vi "Unescape String.vi"(11 "value":string) -> (3 "unescaped string":string)   [LabVIEW 2017, in "LVJSON.lvlib" / "JSON String.lvclass"]
uses:
  JSON String.lvclass
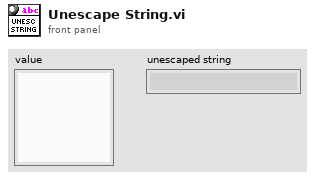
[diagram p1: front panel]
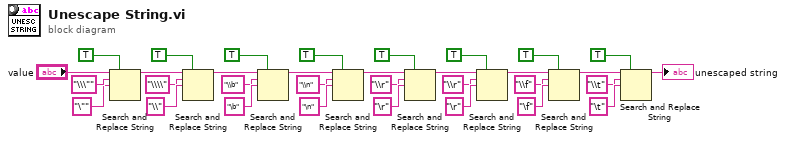
[diagram p0: block diagram]
diagram:
  n1 = Search and Replace String(replace all?=TRUE ("replace all? (F)"), input string="value", search string="\\\"" ("replace string (\"\")"), replace string="\"" ("search string")) -> (result string=w23:string)  [unwired: 4 in, 3 out]
  n2 = Search and Replace String(replace all?=TRUE ("replace all? (F)"), input string=w23, search string="\\\\" ("replace string (\"\")"), replace string="\\" ("search string")) -> (result string=w22:string)  [unwired: 4 in, 3 out]
  n3 = Search and Replace String(replace all?=TRUE ("replace all? (F)"), input string=w22, search string="\\b" ("replace string (\"\")"), replace string="\b" ("search string")) -> (result string=w29:string)  [unwired: 4 in, 3 out]
  n4 = Search and Replace String(replace all?=TRUE ("replace all? (F)"), input string=w29, search string="\\n" ("replace string (\"\")"), replace string="\n" ("search string")) -> (result string=w27:string)  [unwired: 4 in, 3 out]
  n5 = Search and Replace String(replace all?=TRUE ("replace all? (F)"), input string=w27, search string="\\r" ("replace string (\"\")"), replace string="\r" ("search string")) -> (result string=w25:string)  [unwired: 4 in, 3 out]
  n6 = Search and Replace String(replace all?=TRUE ("replace all? (F)"), input string=w25, search string="\\r" ("replace string (\"\")"), replace string="\r" ("search string")) -> (result string=w20:string)  [unwired: 4 in, 3 out]
  n7 = Search and Replace String(replace all?=TRUE ("replace all? (F)"), input string=w20, search string="\\f" ("replace string (\"\")"), replace string="\f" ("search string")) -> (result string=w18:string)  [unwired: 4 in, 3 out]
  n8 = Search and Replace String(replace all?=TRUE ("replace all? (F)"), input string=w18, search string="\\t" ("replace string (\"\")"), replace string="\t" ("search string")) -> (result string=→"unescaped string":string)  [unwired: 4 in, 3 out]
